vi "MALT160T set one output.vi"() -> ()   [LabVIEW 2018]
uses:
  <instrlib>/AltonTech MALT/AltonTech MALT200817.lvlib
panel:
  in  "Kn":i32=1
  in  "Address":i32=3 format="%02x"
  in  "Kn":bool
  in  "stop":bool
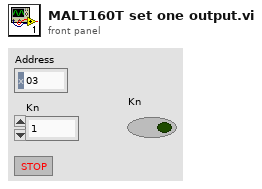
[diagram p1: front panel]
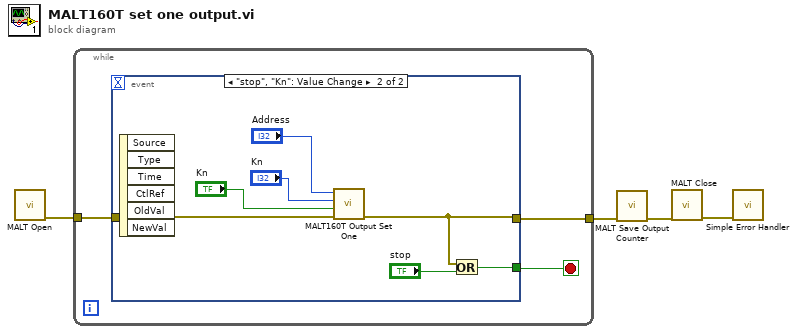
[diagram p0: block diagram]
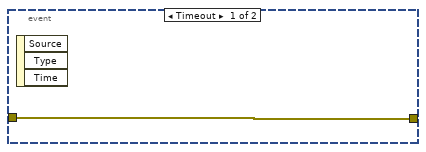
[diagram p2: hidden frame]
diagram:
  n1 = call <instrlib>:"MALT Open.vi"() -> ("error out"=w4:errorcluster)  [unwired: 10 in, 1 out]
  n2 = while {
    tunnel: w4 -> [w7]
    tunnel: [w6] -> w2
    stop <- w5 stop-if-true
    n3 = event shown="[1] \"stop\", \"Kn\": Value Change" {
      selector: _ -> [_ _]
      dyn-events: _ -> [_ _]
      timeout: _ -> [_ _]
      tunnel: w7 -> [w8 w14]
      tunnel: [w8 w13] -> w6
      tunnel: [_ w11] -> w5
      event Timeout {
        n4 = event-data() -> ()  [unwired: 1 in, 3 out]
      }
      event "stop", "Kn": Value Change {
        n5 = event-data() -> ()  [unwired: 1 in, 6 out]
        n6 = call <instrlib>:"MALT160T Output Set One.vi"("error in"=w14, "State"="Kn", "Kn"="Kn", "Address"="Address") -> ("error out"=w13:errorcluster)  [unwired: 7 in]
        n7 = Or(x=w13, y="stop") -> (x .or. y?=w11:bool)
      }
    }
  }
  n8 = call <instrlib>:"MALT Save Output Counter.vi"("error in"=w2) -> ("error out"=w1:errorcluster)  [unwired: 10 in]
  n9 = call <instrlib>:"MALT Close.vi"("error in"=w1) -> ("error out"=w3:errorcluster)  [unwired: 10 in]
  n10 = call <vilib>:"Simple Error Handler.vi"("error in (no error)"=w3) -> ()  [unwired: 4 in, 5 out]
